vi "CHR 62150 DC PS.vi"   [LabVIEW 2018]
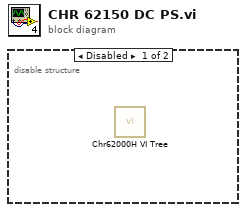
[diagram p0: block diagram]
diagram:
  n1 = disable-structure shown="Disabled" {
    frame Disabled {
      n2 = call <instrlib>:"Chr62000H VI Tree.vi"() -> ()  [unwired: 12 in]
    }
    frame Enabled {
    }
  }
